vi "Configure Module from Switches JSON.vi"() -> ()   [LabVIEW 2017, in "SLSC Switch Examples.lvlib"]
uses:
  SLSC Switch Examples.lvlib
  SLSC Switch/Shared/Endpoint Configuration Cluster.ctl
  SLSC Switch/Shared/Endpoint Configuration Enum.ctl
  NationalInstruments.VeriStand.SystemDefinitionAPI
  SLSC Switch/Scripting/SLSC Switch Scripting.lvlib
  SLSC Switch/Shared/SLSC Switch Shared.lvlib
panel:
  in  "Model":string="SLSC-12251"
  in  "Resource":refnum<k21>
  in  "Slot Number":u32=1
  in  "Switches JSON file":path=path "C:/Program Files (x86)/National Instruments/Shared/NI-SLSC Switch/Modules/SLSC-12251-switches.json"
  in  "Output System Definition file":path
  in  "Input System Definition File":path
  # "Overview: Demonstrates using the SLSC Switch custom device scripting API to configure an instance of the custom device without requiring the hardware be present. By default, the configuration is for an NI SLSC-12251.\nInstructions:\n1. Manually add an instance of the SLSC Switch custom device to a VeriStand system definition. This cannot currently be scripted. \n2. Browse to the system definition file to be used as input.\n3. Browse to a path to save the system definition file as output.\n4. Browse to the JSON file containing the switch definition, typically provided by the vendor.\n5. Select the slot number, model number, and resource/device name to script into the system definition file.\n5. Run the VI and verify its results."
  # "System Definition Files"
  # "Custom Device Configuration"
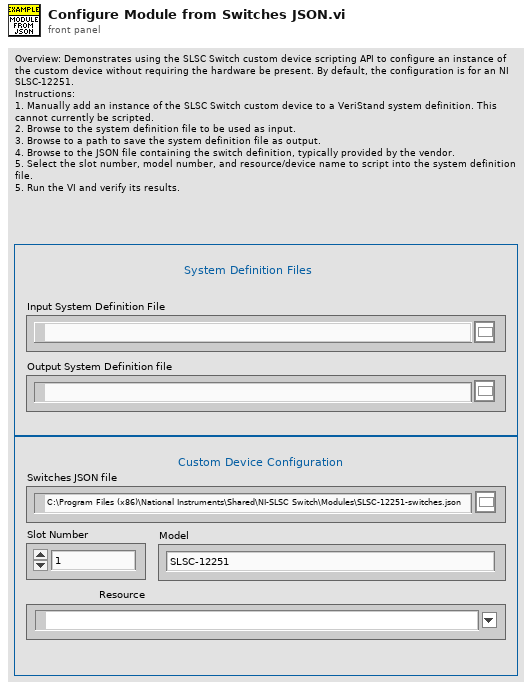
[diagram p1: front panel]
types:
  T1 = typedef "Custom Device API.lvlib/Custom Device Item Ref.ctl" = u64
  T2 = typedef "SLSC Switch Shared.lvlib/Endpoint Configuration Enum.ctl" = enum16{"Load", "Source", "Configuration"}
  T3 = typedef "SLSC Switch Shared.lvlib/Endpoint Configuration Cluster.ctl" = cluster{"Endpoint":string, "Configuration":T2}
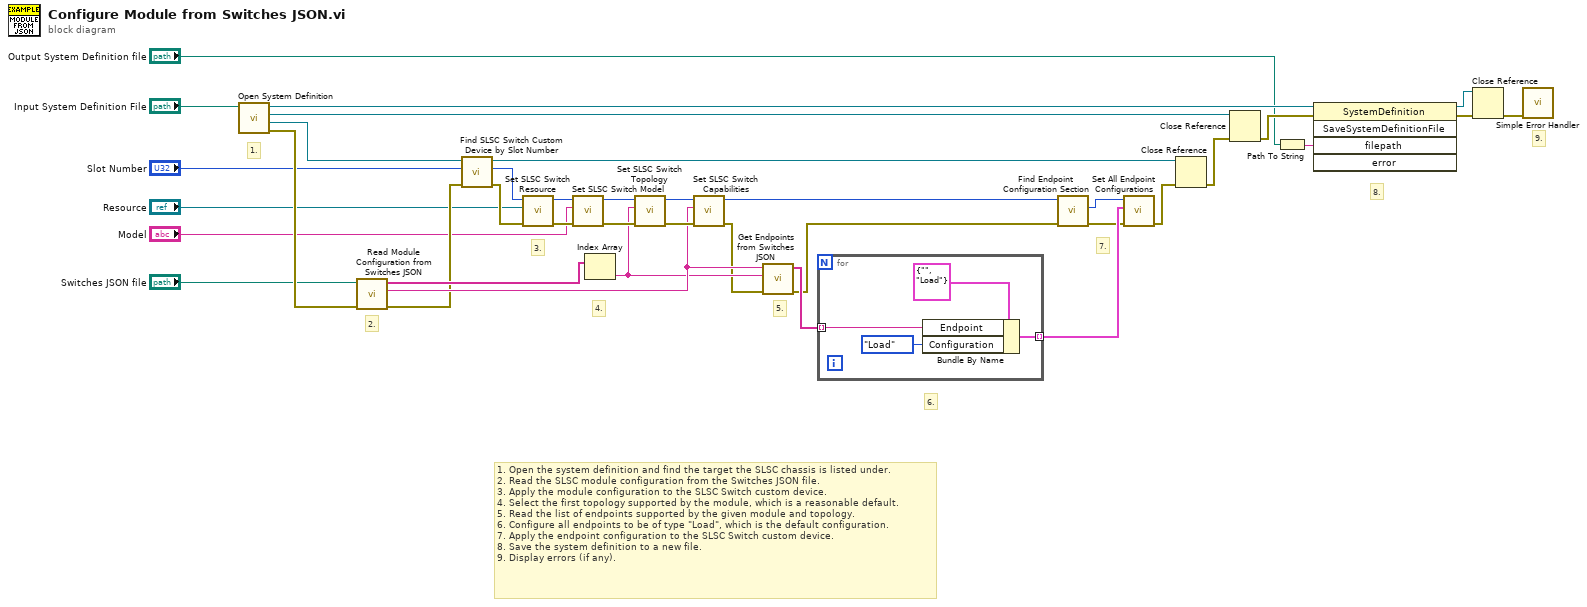
[diagram p0: block diagram]
diagram:
  # "7."
  # "6."
  # "5."
  # "4."
  # "3."
  # "2."
  # "8."
  # "9."
  # "8."
  # "1."
  # "1. Open the system definition and find the target the SLSC chassis is listed under.\n2. Read the SLSC module configuration from the Switches JSON file.\n3. Apply the module configuration to the SLSC Switch custom device.\n4. Select the first topology supported by the module, which is a reasonable default. \n5. Read the list of endpoints supported by the given module and topology.\n6. Configure all endpoints to be of type \"Load\", which is the default configuration.\n7. Apply the endpoint configuration to the SLSC Switch custom device. \n8. Save the system definition to a new file.\n9. Display errors (if any)."
  n1 = call "Open System Definition.vi"("System Definition File"="Input System Definition File") -> ("error out"=w30:errorcluster, "Target Refnum"=w29:refnum<k24>, "Root Refnum"=w33:refnum<k24>, "System Definition Refnum"=w37:refnum<k24>)  [unwired: 7 in]
  n2 = call "Read Module Configuration from Switches JSON.vi"("error in (no error)"=w30, "switches JSON file"="Switches JSON file") -> ("error out"=w4:errorcluster, "switches json"=w15:string, "topologies"=w17:string[])  [unwired: 7 in]
  n3 = call "Find SLSC Switch Custom Device by Slot Number.vi"("error in (no error)"=w4, "slot number"="Slot Number", "Target in"=w29) -> ("error out"=w9:errorcluster, "SLSC Switch Custom Device Ref"=w10:T1, "Target out"=w28:refnum<k24>)  [unwired: 6 in]
  n4 = call "Set SLSC Switch Resource.vi"("error in (no error)"=w9, "Resource"="Resource", "SLSC Switch Custom Device Ref in"=w10) -> ("error out"=w21:errorcluster, "SLSC Switch Custom Device Ref out"=w22:T1)  [unwired: 7 in]
  n5 = call "Set SLSC Switch Model.vi"("error in (no error)"=w21, "Model"="Model", "SLSC Switch Custom Device Ref in"=w22) -> ("error out"=w16:errorcluster, "SLSC Switch Custom Device Ref out"=w20:T1)  [unwired: 7 in]
  n6 = Index Array(array=w17) -> (element=w14:string)  [unwired: 1 in]
  n7 = call "Set SLSC Switch Topology.vi"("error in (no error)"=w16, "Topology"=w14, "SLSC Switch Custom Device Ref in"=w20) -> ("error out"=w18:errorcluster, "SLSC Switch Custom Device Ref out"=w19:T1)  [unwired: 7 in]
  n8 = call "Set SLSC Switch Capabilities.vi"("error in (no error)"=w18, "Capabilities"=w15, "SLSC Switch Custom Device Ref in"=w19) -> ("error out"=w13:errorcluster, "SLSC Switch Custom Device Ref out"=w7:T1)  [unwired: 7 in]
  n9 = call "Get Endpoints from Switches JSON.vi"("error in (no error)"=w13, "topology"=w14, "switches json"=w15) -> ("error out"=w8:errorcluster, "endpoints"=w12:string[])  [unwired: 7 in]
  n10 = for {
    tunnel: w12 -> [w40] mode=indexing
    tunnel: [w38] -> w11 mode=indexing
    n11 = Bundle By Name(cluster=T3 {"Endpoint"="", "Configuration"=enum."Load"} ("All Endpoint Configurations"), "Endpoint"=w40, "Configuration"=Endpoint_Configuration_Enum."Load") -> (w38:T3)
  }
  n12 = call "Find Endpoint Configuration Section.vi"("error in (no error)"=w8, "SLSC Switch Custom Device Ref in"=w7) -> ("error out"=w5:errorcluster, "Endpoint Config Section Ref"=w6:T1)  [unwired: 7 in, 1 out]
  n13 = call "Set All Endpoint Configurations.vi"("error in (no error)"=w5, "All Endpoint Configurations"=w11, "Endpoint Configuration Section Ref in"=w6) -> ("error out"=w26:errorcluster)  [unwired: 7 in, 1 out]
  n14 = Close Reference(reference=w28, error in (no error)=w26) -> (error out=w27:errorcluster)
  n15 = Close Reference(reference=w33, error in (no error)=w27) -> (error out=w32:errorcluster)
  n16 = Path To String(path="Output System Definition file") -> (string=w36:string)
  n17 = invoke class="SystemDefinition" method="SaveSystemDefinitionFile"(reference=w37, error in=w32, "filepath"=w36) -> (reference out=w34:refnum<k24>, error out=w35:errorcluster)  [unwired: 2 in, 3 out]
  n18 = Close Reference(reference=w34, error in (no error)=w35) -> (error out=w25:errorcluster)
  n19 = call <vilib>:"Simple Error Handler.vi"("error in (no error)"=w25) -> ()  [unwired: 1 in, 8 out]
